vi "Calc Slope-Offset and Interpolate.vi"(7 "New x":dbl=3.0, 8 "Second y":dbl=4.0, 9 "First y":dbl=2.0, 10 "Second x":dbl=2.0, 11 "First X":dbl=1.0) -> (2 "Offset":dbl, 3 "Slope":dbl, 5 "New Y":dbl)   [LabVIEW 2010]
doc: "This vi will solve y=mx+b from a pair of XY coordinates, and it will return a new Y value in response to a new X value."
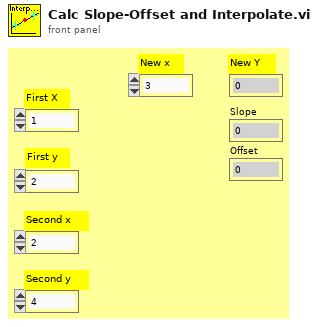
[diagram p1: front panel]
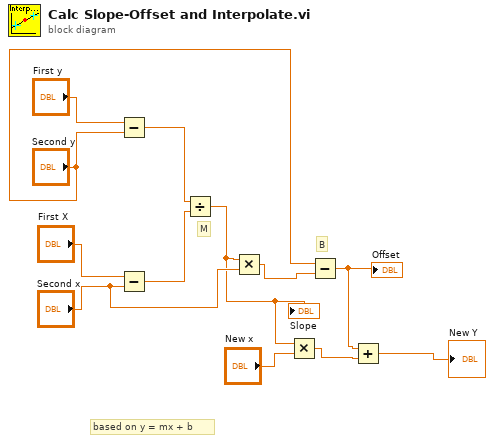
[diagram p0: block diagram]
diagram:
  # "B"
  # "based on y = mx + b"
  # "M"
  n1 = Subtract(x="First y", y="Second y") -> (x-y=w10:dbl)
  n2 = Subtract(x="First X", y="Second x") -> (x-y=w9:dbl)
  n3 = Divide(x=w10, y=w9) -> (x/y=w4:dbl)
  "Slope" <- w4
  n4 = Multiply(x=w4, y="Second x") -> (x*y=w7:dbl)
  n5 = Multiply(x=w4, y="New x") -> (x*y=w3:dbl)
  n6 = Subtract(x="Second y", y=w7) -> (x-y=w2:dbl)
  "Offset" <- w2
  n7 = Add(x=w2, y=w3) -> (x+y=→"New Y":dbl)
